vi "Register gRPC Event.vi"(8 "error in (no error)":errorcluster, 10 "Event Data":refnum<class "ServiceBase.lvclass">) -> (0 "error out":errorcluster)   [LabVIEW 2023, in "Head Worker.lvclass"]
uses:
  Head Worker.lvclass
  <vilib>/gRPC/LabVIEW gRPC Servicer/ServiceBase/ServiceBase.lvclass
panel:
  # "Connector Pane"
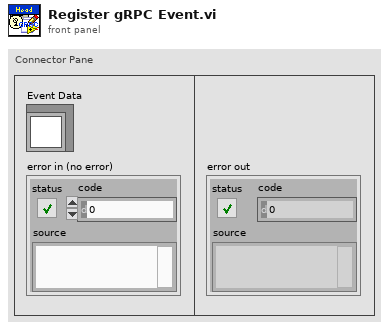
[diagram p1: front panel]
types:
  T1 = typedef "Head Worker.lvclass/Event Data.ctl" = cluster{"gRPC streamAI services":refnum<user-event>, "gRPC Server Stop":refnum<user-event>}
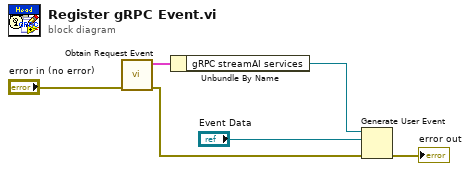
[diagram p0: block diagram]
diagram:
  n1 = call "Obtain Request Event.vi"("error in (no error)"="error in (no error)") -> ("error out"=w3:errorcluster, "output cluster"=w6:T1)  [unwired: 9 in]
  n2 = Unbundle By Name(w6) -> ("gRPC streamAI services"=w5:refnum<user-event>)
  n3 = Generate User Event(user event=w5, event data cluster="Event Data", error in=w3) -> (error out=→"error out":errorcluster)  [unwired: 1 in, 1 out]
